vi "Set Guardian Message SV.vi"(8 "error in (no error)":errorcluster, 9 "Guardian Message":refnum<class "Circus Shared Variables.lvclass">, 10 "ID":string, 11 "Guardian List in":refnum<class "Guardian List.lvclass">) -> (0 "error out":errorcluster, 3 "Guardian List out":refnum<class "Guardian List.lvclass">)   [LabVIEW 2020, in "TALOS.lvlib" / "Classes.lvlib" / "Guardian List.lvclass"]
uses:
  Guardian List.lvclass
  Circus Shared Variables/Circus Shared Variables.lvclass
  Guardian List.lvclass/Guardian List.ctl
  Ancestor/Ancestor/Ancestor.lvclass/Ancestor.ctl
  FGV/Error Memory/Get Error Description.vi
  Support VIs/Get PC name.vi
  Ancestor/Ancestor/Read ID.vi
  Support VIs/Get Class Name.vi
  <vilib>/Utility/error.llb/Clear Errors.vi
  FGV/Error Memory/Error Memory Core.vi
  <vilib>/AdvancedString/Delimited String to 1D String Array.vi
  Support VIs/Circus Root Path.vi
  FGV/Error Memory/Error Crt Lvl checker.vi
  FGV/Error Memory/Error Memory Core.vi/40c8088d-b597-4017-91af-faa98e00292e.vi
  FGV/Error Memory/Error Memory Core.vi/d4a3ab98-063c-4e44-b43d-fbdcfe6c2be2.vi
  Support VIs/Global Memory.vi
  <vilib>/Utility/LVClass/Get LV Class Name.vi
  Support VIs/Is in Packed Library.vi
  Support VIs/TALOS Root path.vi
  Support VIs/Read CSV worksheet.vi
  Support VIs/Global Constants.vi
  <vilib>/Utility/error.llb/General Error Handler.vi
  Ancestor/Ancestor/Ancestor.lvclass
  <vilib>/Comparison/Equal/Equal Functor/Equal Functor.lvclass
  TALOS.lvlib
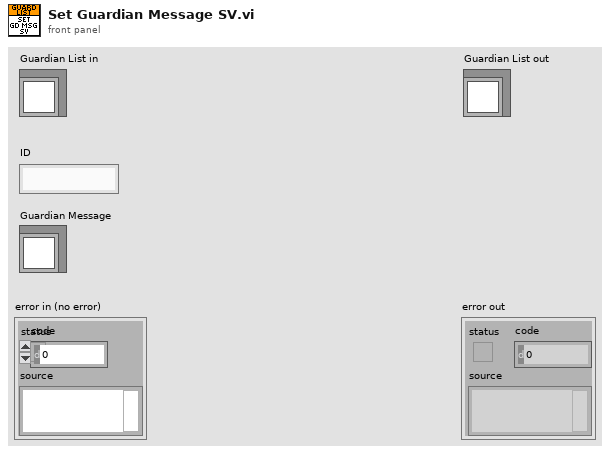
[diagram p1: front panel]
types:
  T1 = typedef "TALOS.lvlib/Classes.lvlib/Guardian List.lvclass/Guardian Properties.ctl" = cluster{"Alive":bool, "Last Seen":timestamp, "Guardian Message":refnum<class "Circus Shared Variables.lvclass">, "IP":string, "TCP Writer associated ID":string, "uS List received":bool, "Abort":bool, "Bearer":bool}
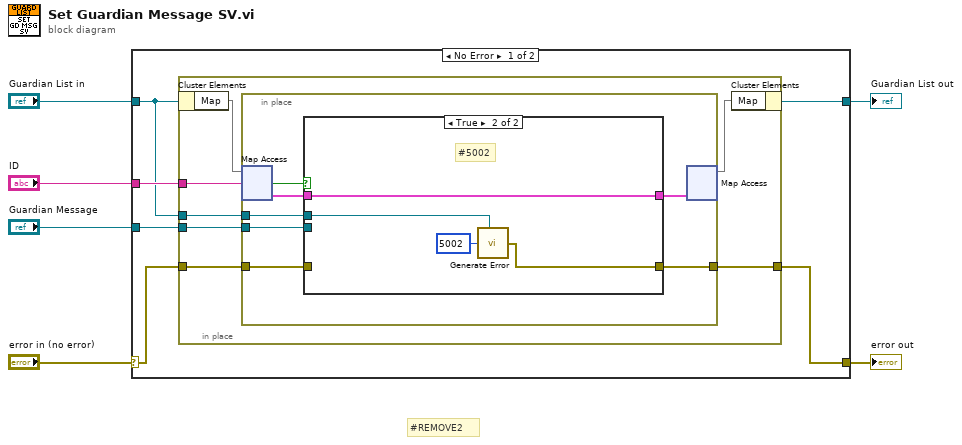
[diagram p0: block diagram]
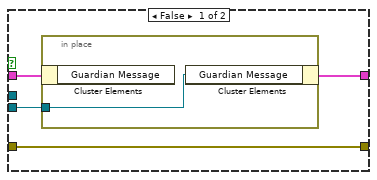
[diagram p2: hidden frame]
diagram:
  # "#REMOVE2"
  n1 = case shown="No Error" "error in (no error)" {
    selector: "error in (no error)" -> [w8 w37]
    tunnel: [w7 w37] -> w5
    tunnel: [w11 w36] -> w3
    tunnel: "Guardian List in" -> [w9 w36]
    tunnel: "ID" -> [w12 _]
    tunnel: "Guardian Message" -> [w10 _]
    frame No Error {
      n2 = in-place {
        in-place-border: w12 -> [w19]
        in-place-border: w10 -> [w16]
        in-place-border: w9 -> [w15]
        in-place-border: w8 -> [w14]
        in-place-border: [w13] -> w7
        n3 = in-place-cluster #1(w9) -> ("Map"=w18:map{string, T1})
        n4 = in-place {
          in-place-border: w16 -> [w24]
          in-place-border: w15 -> [w20]
          in-place-border: w14 -> [w22]
          in-place-border: [w21] -> w13
          n5 = in-place-map #2(w18, w19) -> (w26:T1, w23:bool)  [unwired: 1 in]
          n6 = case shown="True" w23 {
            tunnel: w26 -> [w30 w35]
            tunnel: [w29 w35] -> w25
            tunnel: w24 -> [w28 _]
            tunnel: w22 -> [w27 _]
            tunnel: [w27 w34] -> w21
            tunnel: w20 -> [_ w33]
            frame False {
              n7 = in-place {
                in-place-border: w28 -> [w31]
                n8 = in-place-cluster #3(w30) -> ()  [unwired: 1 out]
                n9 = in-place-cluster #3("Guardian Message"=w31) -> (w29:T1)
              }
            }
            frame True {
              # "#5002"
              n10 = call "Generate Error.vi"("Class"=w33, "Error Code"=5002) -> ("error out"=w34:errorcluster)  [unwired: 5 in]
            }
          }
          n11 = in-place-map #2(w25) -> (w17:map{string, T1})  [unwired: 1 in, 2 out]
        }
        n12 = in-place-cluster #1("Map"=w17) -> (w11:refnum<class "Guardian List.lvclass">)
      }
    }
    frame Error {
    }
  }
  "error out" <- w5
  "Guardian List out" <- w3
